vi "Print Outside Range Message.vi"(7 "Message Type":T2=enum."Error", 8 "error in (no error)":errorcluster, 11 "Message Values":T1) -> ()   [LabVIEW 2014, in "Waveform Analog Output Engine.lvlib"]
uses:
  Waveform Analog Output Engine.lvlib
  Console Message Type.ctl
  <vilib>/NI Veristand/Custom Device Tools/Custom Device Utility Library/Custom Device Utility Library.lvlib
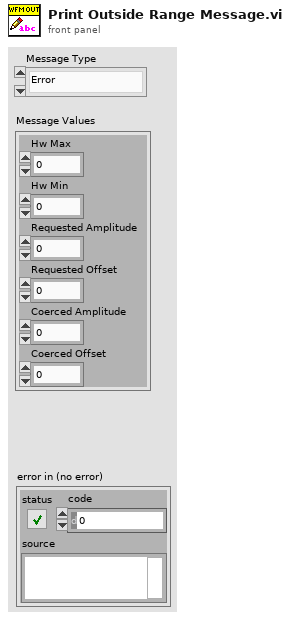
[diagram p1: front panel]
types:
  T1 = cluster{"Hw Max":dbl, "Hw Min":dbl, "Requested Amplitude":dbl, "Requested Offset":dbl, "Coerced Amplitude":dbl, "Coerced Offset":dbl}
  T2 = typedef "Waveform Analog Output Engine.lvlib/Console Message Type.ctl" = enum16{"Range Warning", "Error"}
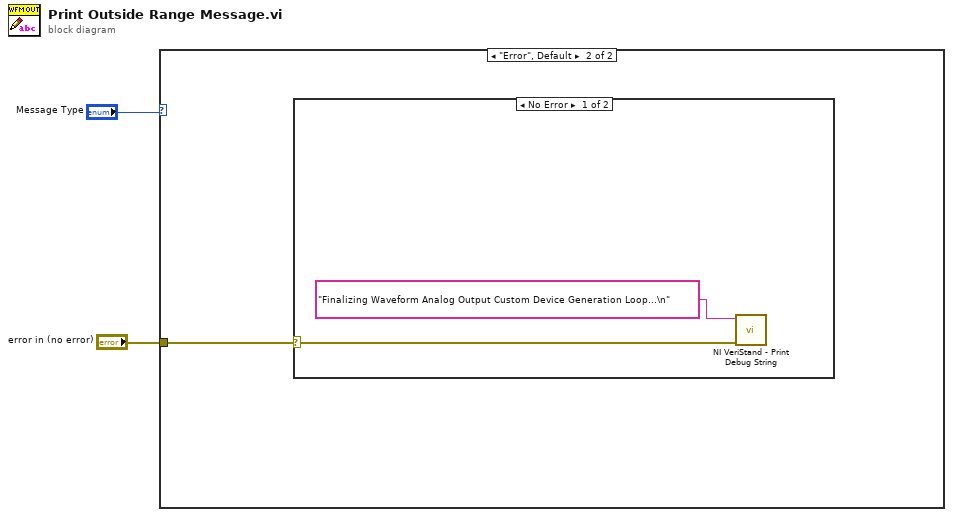
[diagram p0: block diagram]
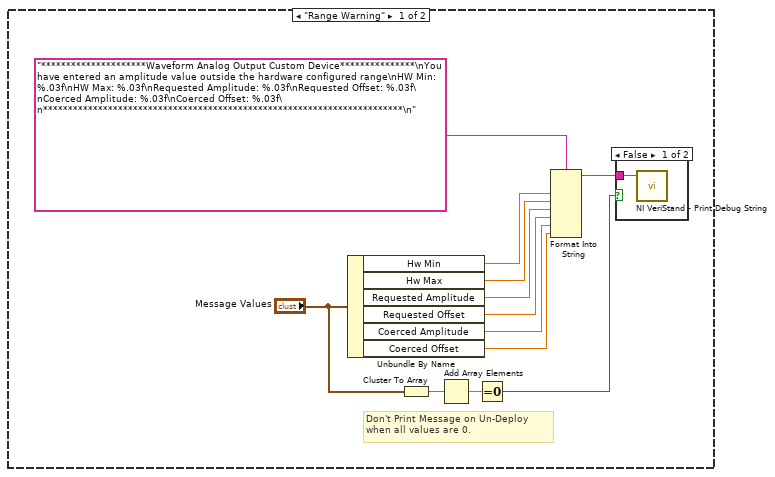
[diagram p2: hidden frame]
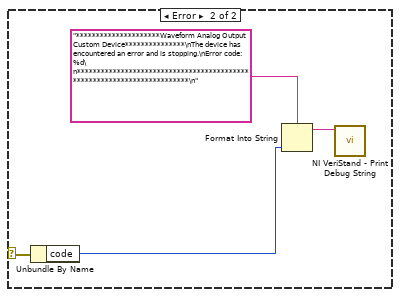
[diagram p4: hidden frame]
diagram:
  n1 = case shown="\"Error\", Default" "Message Type" {
    tunnel: "error in (no error)" -> [_ w16]
    frame "Range Warning" {
      # "Don't Print Message on Un-Deploy \nwhen all values are 0."
      n2 = Unbundle By Name("Message Values") -> ("Hw Min"=w8:dbl, "Hw Max"=w7:dbl, "Requested Amplitude"=w12:dbl, "Requested Offset"=w11:dbl, "Coerced Amplitude"=w10:dbl, "Coerced Offset"=w9:dbl)
      n3 = Cluster To Array(cluster="Message Values") -> (array=w5:dbl[])
      n4 = Add Array Elements(numeric array=w5) -> (sum=w4:dbl)
      n5 = Equal To 0?(x=w4) -> (x = 0?=w3:bool)
      n6 = Format Into String(format string="*********************Waveform Analog Output Custom Device***************\nYou have entered an amplitude value outside the hardware configured range\nHW Min: %.03f\nHW Max: %.03f\nRequested Amplitude: %.03f\nRequested Offset: %.03f\nCoerced Amplitude: %.03f\nCoerced Offset: %.03f\n************************************************************************\n", w8, w7, w12, w11, w10, w9) -> (resulting string=w13:string)  [unwired: 2 in, 1 out]
      n7 = case shown="False" w3 {
        tunnel: w13 -> [w15 _]
        frame False {
          n8 = call <vilib>:"NI VeriStand - Print Debug String.vi"("Message"=w15) -> ()  [unwired: 10 in, 1 out]
        }
        frame True {
        }
      }
    }
    frame "Error", Default {
      n9 = case shown="No Error" w16 {
        selector: w16 -> [w17 w22]
        frame No Error {
          n10 = call <vilib>:"NI VeriStand - Print Debug String.vi"("error in (no error)"=w17, "Message"="Finalizing Waveform Analog Output Custom Device Generation Loop...\n") -> ()  [unwired: 9 in, 1 out]
        }
        frame Error {
          n11 = Unbundle By Name(w22) -> ("code"=w21:i32)
          n12 = Format Into String(format string="*********************Waveform Analog Output Custom Device***************\nThe device has encountered an error and is stopping.\nError code: %d\n************************************************************************\n", w21) -> (resulting string=w20:string)  [unwired: 2 in, 1 out]
          n13 = call <vilib>:"NI VeriStand - Print Debug String.vi"("Message"=w20) -> ()  [unwired: 10 in, 1 out]
        }
      }
    }
  }
